vi "RADAR (Host).vi"() -> ()   [LabVIEW 2017]
uses:
  <vilib>/userdefined/Silver/nirio_resource_slv.ctl
  <vilib>/Utility/error.llb/DialogType.ctl
  <vilib>/rvi/interface/RandomDataEmulation/nirviRandomDataOpen.vi
  <vilib>/rvi/interface/common/niFpgaCacheSessionInfoDynamic.vi
  <vilib>/FPGAPlugInAG/Dynamic/niLvFpga_Close_Dynamic.vi
  <vilib>/rvi/interface/nirviOpenFPGA/nirviOpenFPGA.xnode
  FPGA/RADAR (NI 5791 FPGA).vi
  <vilib>/rvi/interface/nirviCloseFPGA/nirviCloseFPGA.xnode
panel:
  in  "Select Wave":u8
  in  "Guard width (us)":dbl=1.076923076923077 format="%#_10g"
  in  "nroCpi":u32=1
  in  "CPI":u32=4
  in  "Stop":bool
  in  "PRP (ms)":dbl=0.01076923
  in  "Pulse width (us)":dbl=1.076923076923077 format="%#_10g"
  in  "Beta":fxp<+,32,32> format="%.0pHz"
  in  "Oversampling factor":u8=1
  in  "cte Q":i16
  in  "cte I":i16=10000
  in  "RIO Device":T1="RIO0"
  in  "LO frequency [Hz]":dbl=-1.0 caption="LO Frequency [Hz]" format="%#.3pHz"
  in  "frequency [Hz]":dbl=2450000000.0 caption="Frequency [Hz]" format="%#.3pHz"
  in  "clock source":string(combo)="Internal" caption="Clock Source"
  in  "reference clock source":string(combo)="Internal" caption="Reference Clock Source"
  in  "sample rate [S/s]":dbl=130000000.0 caption="Sample Rate [S/s]" format="%#.3pS/s"
  in  "reference level [dBm]":dbl=-10.0 caption="Reference Level [dBm]" format="%#_gdBm"
  in  "Tab Control":T2(tab)
  out "Rx Power Level":dbl[](graph) caption="Power Level"
  out "Rx Power Spectrum":cluster{"f0":dbl, "df":dbl, "magnitude":dbl[]}(graph) caption="Power Spectrum"
  out "Rx I & Q Data":dbl[][](graph) caption="I & Q Data"
  # "Streaming"
  # "This template is for the NI-579X Streaming design, a design that shows the basics of streaming data from a NI-579X device.\n\nSee the block diagram for more information on how to use this template."
  # "Tx Generation Engine"
  # "Case 0: constants (I/Q)\nCase 1: Chirp (I/Q) Generation Panel \nCase 2: Barker 7 code (I: +1,+1,+1,-1,-1,+1,-1 / Q: 0)\nCase 3: Barker 13 code (I: +1,+1,+1,+1,+1,-1,-1,+1,+1,-1,+1,-1,+1 / Q: 0)"
  # "Constant Wave Generation"
  # "Chirp Wave Generation"
  # "Barker Wave Generation"
  # "Clock Configuration"
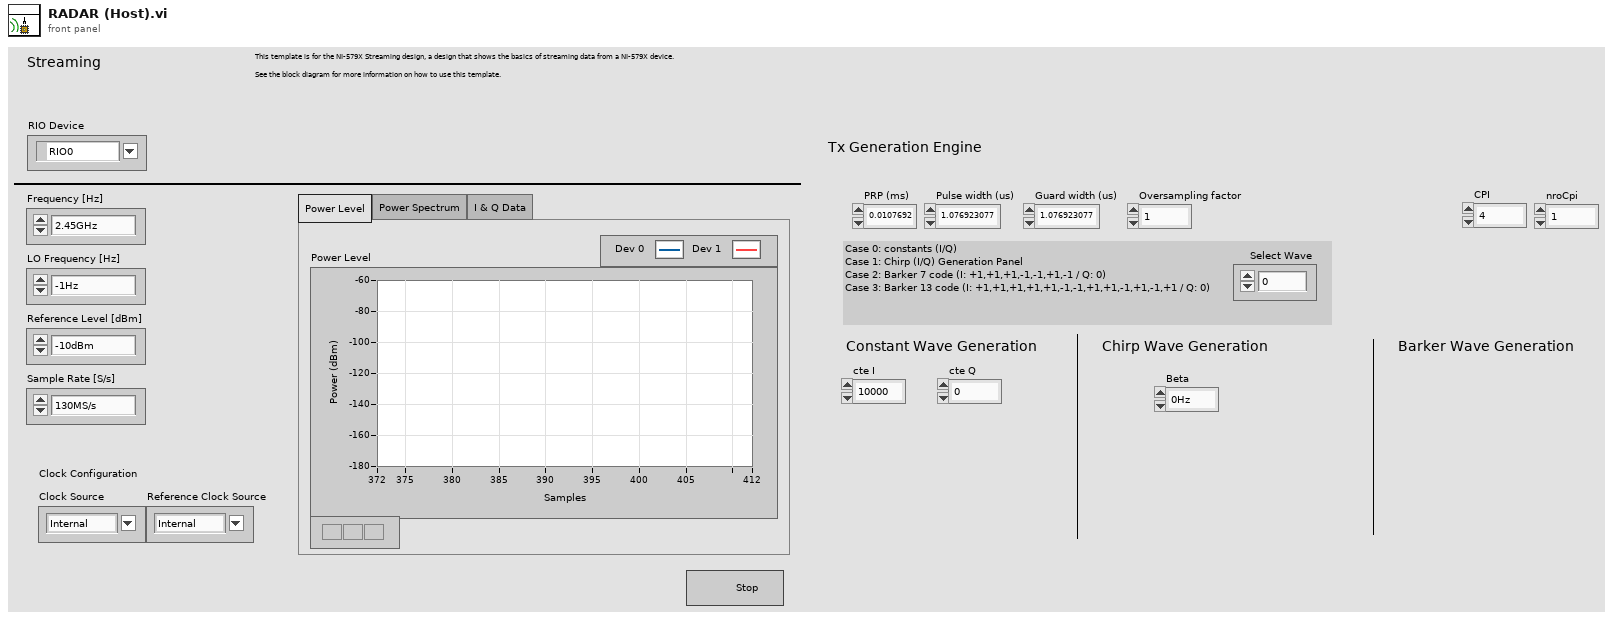
[diagram p1: front panel]
types:
  T1 = typedef "nirio_resource_slv.ctl" = tag
  T2 = enum32{"Power Level", "Power Spectrum", "I & Q Data"}
  T3 = typedef "DialogType.ctl" = u16
  T4 = typedef "niInstr Register Bus v0 Host.lvlib/Register Bus Session.ctl" = refnum<queue>
  T5 = cluster{dbl, dbl, "PRP (ms)":dbl, "Pulse width (us)":dbl, dbl, "frequency [Hz]":dbl, "reference level [dBm]":dbl, dbl, dbl, dbl, dbl, "Guard width (us)":dbl}
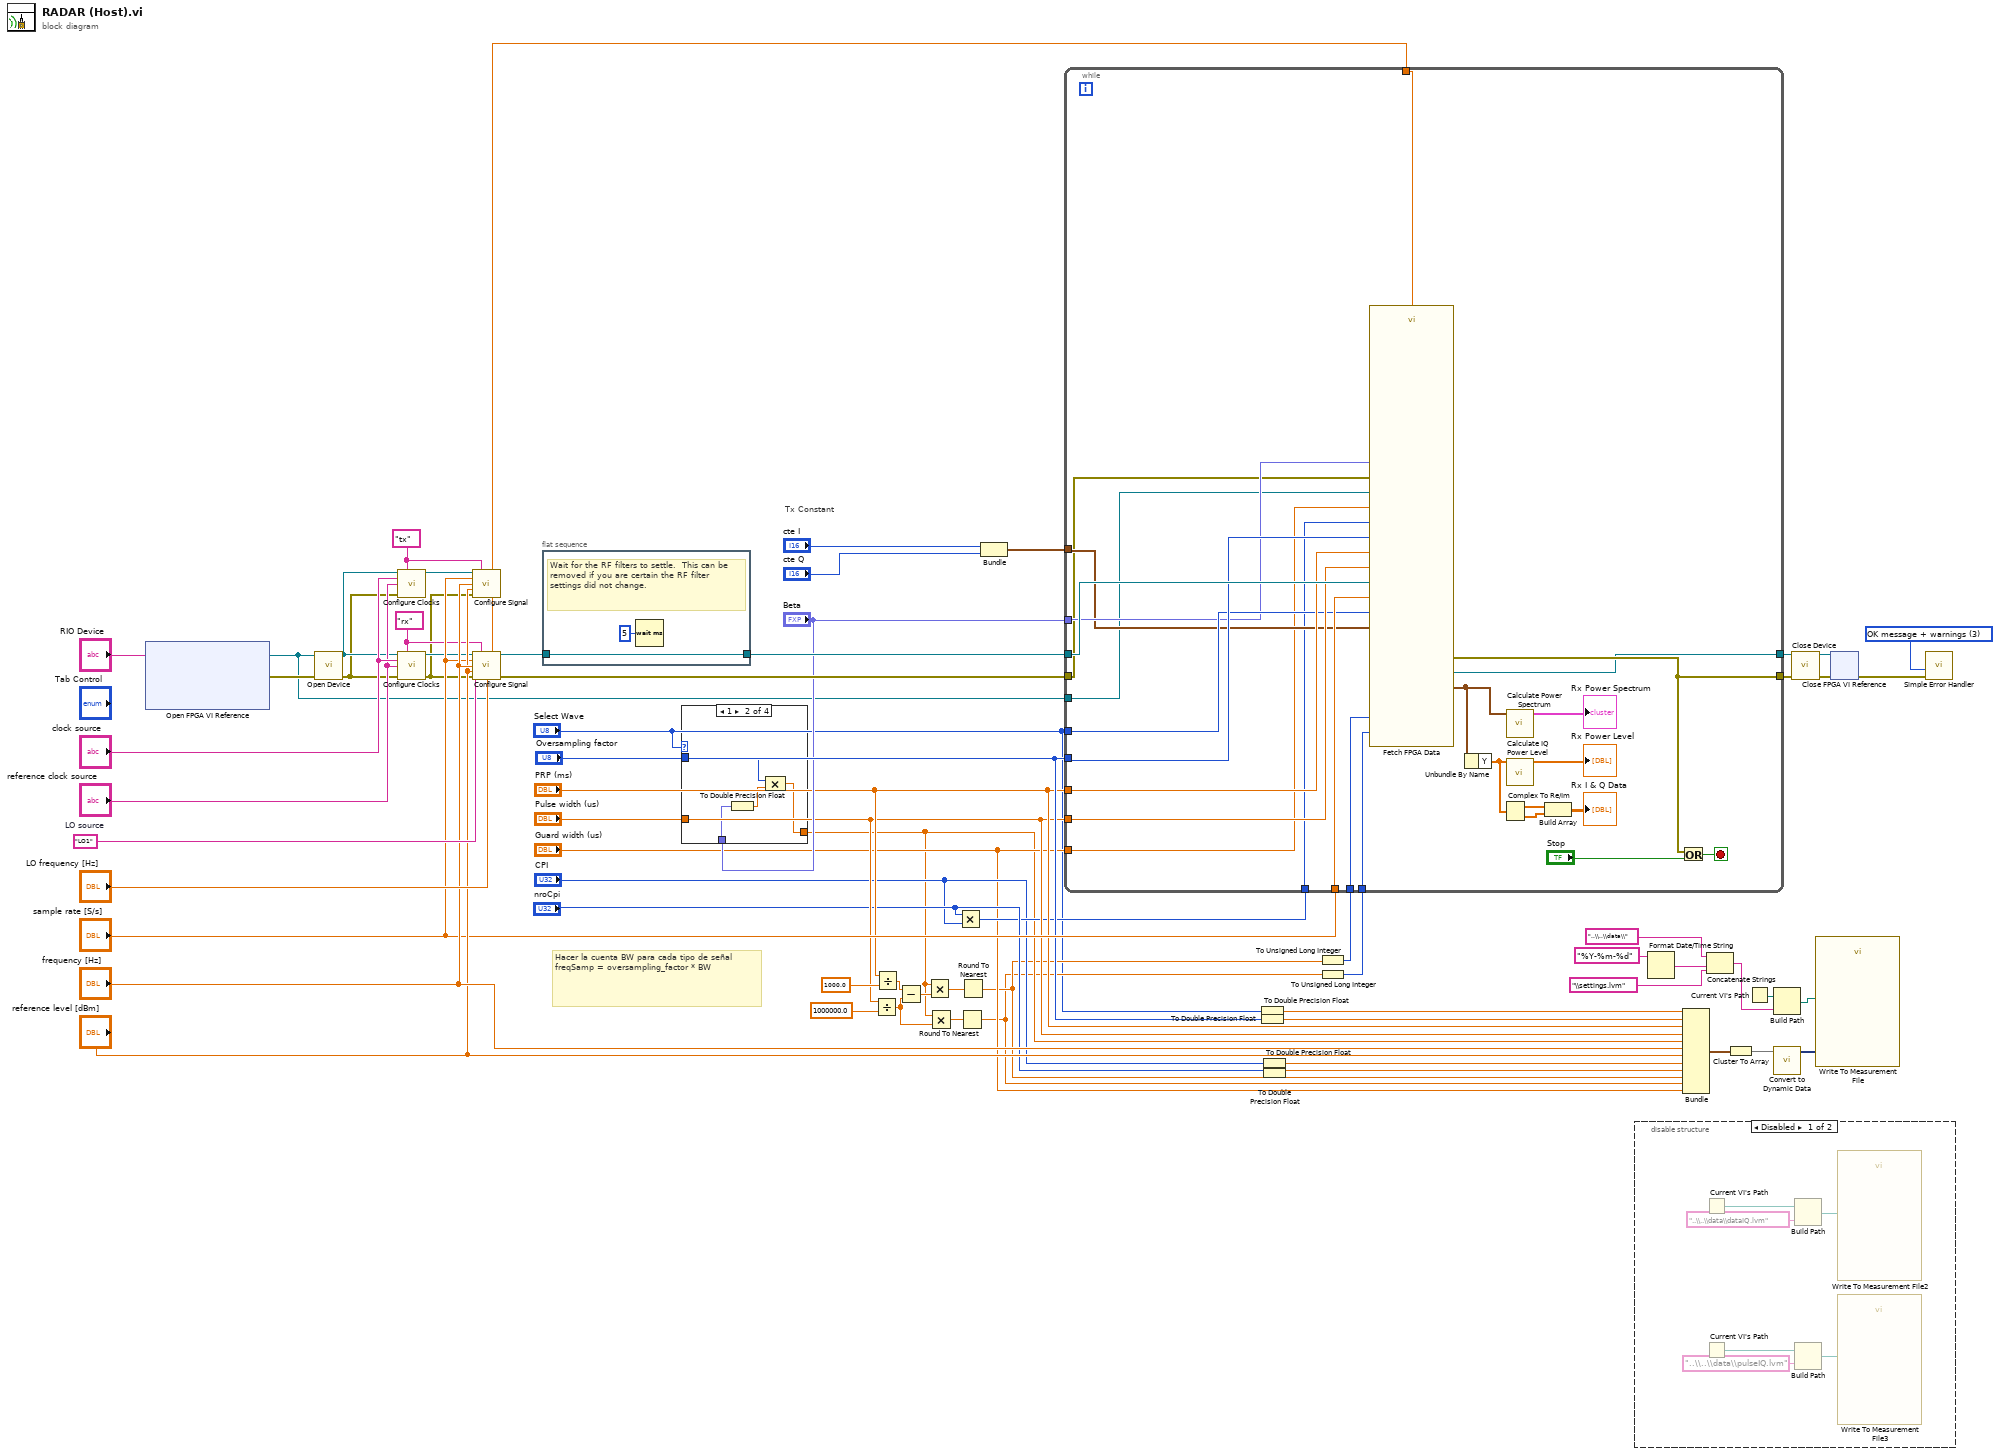
[diagram p0: block diagram]
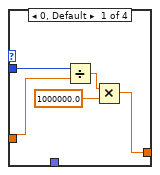
[diagram p3: hidden frame]
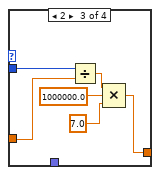
[diagram p4: hidden frame]
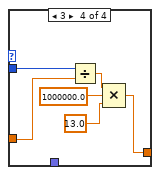
[diagram p5: hidden frame]
diagram:
  w4 = "tx" ("scope")
  w7 = "rx" ("scope")
  w63 = "LO1"  # LO source
  w65 = T3 3 items=["no dialog", "OK message", "continue or stop message", "OK message + warnings", "continue/stop + warnings"] ("type of dialog (OK msg:1)")
  # "Tx Constant"
  # "Hacer la cuenta BW para cada tipo de señal\nfreqSamp = oversampling_factor * BW"
  n1 = xnode "Open FPGA VI Reference"("resource name"="RIO Device") -> ("FPGA VI Reference Out"=w1:refnum<k20>, "error out"=w61:errorcluster)  [unwired: 1 in]
  n2 = call "Open Device.vi"("fpga ref"=w1, "error in"=w61) -> ("Register Bus (out)"=w3:T4, "error out"=w2:errorcluster)  [unwired: 12 in]
  n3 = call "Configure Clocks.vi"("Register Bus"=w3, "scope"=w4, "clock source"="clock source", "reference clock source"="reference clock source", "error in"=w2) -> ("Register Bus (out)"=w6:T4)  [unwired: 9 in, 1 out]
  n4 = call "Configure Clocks.vi"("Register Bus"=w3, "scope"=w7, "clock source"="clock source", "reference clock source"="reference clock source", "error in"=w2) -> ("Register Bus (out)"=w8:T4, "error out"=w5:errorcluster)  [unwired: 9 in]
  n5 = call "Configure Signal.vi"("Register Bus"=w6, "scope"=w4, "sample rate [S/s]"="sample rate [S/s]", "frequency [Hz]"="frequency [Hz]", "level [dBm]"="reference level [dBm]", "error in"=w5) -> ()  [unwired: 3 in, 7 out]
  n6 = call "Configure Signal.vi"("Register Bus"=w8, "scope"=w7, "sample rate [S/s]"="sample rate [S/s]", "frequency [Hz]"="frequency [Hz]", "level [dBm]"="reference level [dBm]", "error in"=w5, "LO source"=w63, "LO frequency [Hz]"="LO frequency [Hz]") -> ("coerced vertical range [Vpp]"=w57:dbl, "Register Bus (out)"=w56:T4, "error out"=w55:errorcluster)  [unwired: 1 in, 4 out]
  n7 = flat-sequence {
    tunnel: w56 -> [w66]
    tunnel: [w66] -> w64
    frame #0 {
      # "Wait for the RF filters to settle.  This can be removed if you are certain the RF filter settings did not change."
      n8 = Wait (ms)(milliseconds to wait=u32 5) -> ()  [unwired: 1 out]
    }
  }
  n9 = case shown="1" "Select Wave" {
    tunnel: "Oversampling factor" -> [w70 w73 w79 w85]
    tunnel: "Pulse width (us)" -> [w69 _ w80 w86]
    tunnel: [w68 w76 w78 w84] -> w18
    tunnel: "Beta" -> [_ w75 _ _]
    frame 0, Default {
      n10 = Divide(x=w70, y=w69) -> (x/y=w72:dbl)
      n11 = Multiply(x=w72, y=1000000.0) -> (x*y=w68:dbl)
    }
    frame 1 {
      n12 = To Double Precision Float(number=w75) -> (double precision float=w74:dbl)
      n13 = Compound Arithmetic op=MULTIPLY(w73, w74) -> (w76:dbl)
    }
    frame 2 {
      n14 = Divide(x=w79, y=w80) -> (x/y=w82:dbl)
      n15 = Compound Arithmetic op=MULTIPLY(w82, 1000000.0 ("y"), 7.0 ("y")) -> (w78:dbl)
    }
    frame 3 {
      n16 = Divide(x=w85, y=w86) -> (x/y=w88:dbl)
      n17 = Compound Arithmetic op=MULTIPLY(w88, 1000000.0 ("y"), 13.0 ("y")) -> (w84:dbl)
    }
  }
  n18 = Divide(x="Pulse width (us)", y=1000000.0) -> (x/y=w17:dbl)
  n19 = Divide(x="PRP (ms)", y=1000.0) -> (x/y=w31:dbl)
  n20 = Subtract(x=w31, y=w17) -> (x-y=w30:dbl)
  n21 = Multiply(x=w18, y=w30) -> (x*y=w13:dbl)
  n22 = Multiply(x=w18, y=w17) -> (x*y=w12:dbl)
  n23 = Multiply(x="nroCpi", y="CPI") -> (x*y=w28:u32)
  n24 = Round To Nearest(number=w12) -> (nearest integer value=w11:dbl)
  n25 = Round To Nearest(number=w13) -> (nearest integer value=w14:dbl)
  n26 = Bundle("cte I"="cte I", "cte Q"="cte Q") -> (w37:cluster{"cte I":i16, "cte Q":i16})  [unwired: 1 in]
  n27 = To Double Precision Float(number="Select Wave") -> (double precision float=w9:dbl)
  n28 = To Double Precision Float(number="Oversampling factor") -> (double precision float=w46:dbl)
  n29 = To Double Precision Float(number="CPI") -> (double precision float=w43:dbl)
  n30 = To Double Precision Float(number="nroCpi") -> (double precision float=w36:dbl)
  n31 = To Unsigned Long Integer(number=w14) -> (unsigned 32bit integer=w15:u32)
  n32 = To Unsigned Long Integer(number=w11) -> (unsigned 32bit integer=w16:u32)
  n33 = while {
    tunnel: w64 -> [w107]
    tunnel: [w104] -> w52
    tunnel: w57 -> [w106]
    tunnel: "sample rate [S/s]" -> [w102]
    tunnel: w55 -> [w90]
    tunnel: [w105] -> w51
    tunnel: w1 -> [w93]
    tunnel: "PRP (ms)" -> [w100]
    tunnel: "Pulse width (us)" -> [w99]
    tunnel: "Oversampling factor" -> [w98]
    tunnel: "Select Wave" -> [w97]
    tunnel: "Beta" -> [w96]
    tunnel: w37 -> [w95]
    tunnel: w28 -> [w94]
    tunnel: "Guard width (us)" -> [w92]
    tunnel: w15 -> [w91]
    tunnel: w16 -> [w89]
    stop <- w114 stop-if-true
    # "Acquire and Fetch a waveform"
    n34 = call "Fetch FPGA Data.vi"("Register Bus"=w107, "Tx Constant"=w95, "Beta"=w96, "error in"=w90, "Select Wave"=w97, "vertical range [Vpp]"=w106, "PRP (ms)"=w100, "sample rate [S/s]"=w102, "Pulse width (us)"=w99, "Guard width (us)"=w92, "Oversampling factor"=w98, "FPGA VI Reference In"=w93, "nroCPI x CPI"=w94, "numRange"=w91, "pulseRange"=w89) -> ("Register Bus (out)"=w104:T4, "Rx Waveform (CDB WDT)"=w103:waveform(cdb), "error out"=w105:errorcluster)  [unwired: 9 in, 1 out]
    n35 = Unbundle By Name(w103) -> ("Y"=w110:cdb[])
    n36 = Complex To Re/Im(x + iy=w110) -> (x=w109:dbl[], y=w108:dbl[])
    n37 = call "Calculate Power Spectrum.vi"("IQ Waveform"=w103) -> ("power spectrum (dBm)"=→"Rx Power Spectrum":cluster{"f0":dbl, "df":dbl, "magnitude":dbl[]})  [unwired: 14 in]
    n38 = call "Calculate IQ Power Level.vi"("IQ data"=w110) -> ("power level (dBm)"=→"Rx Power Level":dbl[])  [unwired: 14 in]
    n39 = Build Array(w109, w108) -> (→"Rx I & Q Data":dbl[][])
    n40 = Or(x=w105, y="Stop") -> (x .or. y?=w114:bool)
  }
  n41 = disable-structure shown="Disabled" {
    frame Disabled {
      n42 = Current VI's Path() -> (path=w119:path)
      n43 = Current VI's Path() -> (path=w116:path)
      n44 = Build Path(base path=w119, name or relative path="..\\..\\data\\dataIQ.lvm") -> (appended path=w118:path)
      n45 = Build Path(base path=w116, name or relative path="..\\..\\data\\pulseIQ.lvm") -> (appended path=w117:path)
      n46 = call "Write To Measurement File2"("Filename"=w118) -> ()  [unwired: 16 in, 3 out]
      n47 = call "Write To Measurement File3"("Filename"=w117) -> ()  [unwired: 16 in, 3 out]
    }
    frame Enabled {
    }
  }
  n48 = Format Date/Time String(time format string (%c)="%Y-%m-%d") -> (date/time string=w23:string)  [unwired: 2 in]
  n49 = Bundle(w9, w46, "PRP (ms)"="PRP (ms)", "Pulse width (us)"="Pulse width (us)", w18, "frequency [Hz]"="frequency [Hz]", "reference level [dBm]"="reference level [dBm]", w43, w36, w14, w11, "Guard width (us)"="Guard width (us)") -> (w48:T5)  [unwired: 1 in]
  n50 = Concatenate Strings("..\\..\\data\\" ("name or relative path"), w23, "\\settings.lvm" ("name or relative path")) -> (w20:string)
  n51 = Cluster To Array(cluster=w48) -> (array=w47:dbl[])
  n52 = Current VI's Path() -> (path=w27:path)
  n53 = Build Path(base path=w27, name or relative path=w20) -> (appended path=w26:path)
  n54 = call "Convert to Dynamic Data"("Array"=w47) -> ("Dynamic Data Type"=w44:dynamicdata)  [unwired: 3 in]
  n55 = call "Close Device.vi"("Register Bus"=w52, "error in"=w51) -> ("fpga ref"=w58:refnum<k20>, "error out"=w59:errorcluster)  [unwired: 12 in]
  n56 = call "Write To Measurement File"("Signals"=w44, "Filename"=w26) -> ()  [unwired: 15 in, 3 out]
  n57 = xnode "Close FPGA VI Reference"("FPGA VI Reference In"=w58, "error in"=w59) -> ("error out"=w45:errorcluster)
  n58 = call <vilib>:"Simple Error Handler.vi"("type of dialog (OK msg:1)"=w65, "error in (no error)"=w45) -> ()  [unwired: 3 in, 5 out]
